vi "waveform relative time.vi"(8 "error in (no error)":errorcluster, 11 "signal in":waveform(dbl)) -> (0 "error out":errorcluster, 1 "start time":timestamp, 2 "Y":dbl[](array[numeric]), 3 "Relative Time":dbl[](array[numeric]))   [LabVIEW 2022 SP3]
doc: "Get information from waveform."
uses:
  <vilib>/Waveform/WDTOps.llb/WDT Get Waveform Time Array DBL.vi
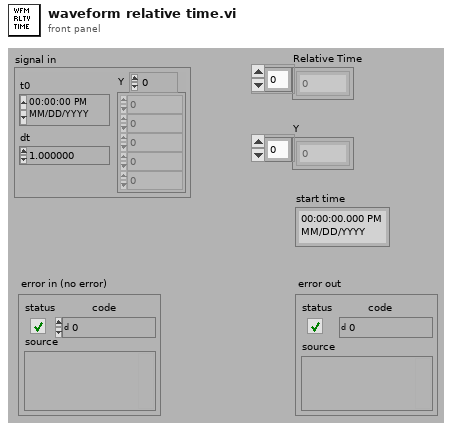
[diagram p1: front panel]
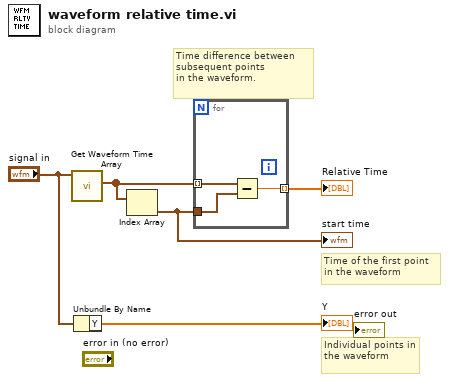
[diagram p0: block diagram]
diagram:
  # "Time of the first point\nin the waveform"
  # "Individual points in the waveform"
  # "Time difference between subsequent points\nin the waveform."
  n1 = call-poly <vilib>:"Get Waveform Time Array.vi"("waveform in"="signal in") -> ("X array"=w1:timestamp[])  [unwired: 9 in, 1 out]
  n2 = Unbundle By Name("signal in") -> ("Y"=→"Y":dbl[])
  n3 = Index Array(array=w1) -> (element=w2:timestamp)  [unwired: 1 in]
  "start time" <- w2
  n4 = for {
    tunnel: w1 -> [w7] mode=indexing
    tunnel: w2 -> [w8]
    tunnel: [w6] -> w3 mode=indexing
    n5 = Subtract(x=w7, y=w8) -> (x-y=w6:dbl)
  }
  "Relative Time" <- w3
